vi "parse_dictionary_to_csv_string.vi"(8 "error in (no error)":errorcluster, 11 "Localization":T1) -> (0 "error out":errorcluster, 3 "CSV String":string)   [LabVIEW 2019]
uses:
  Dictionary--Cluster.ctl
  Font -- Cluster.ctl
  Phrase Dictionary Entry -- Cluster.ctl
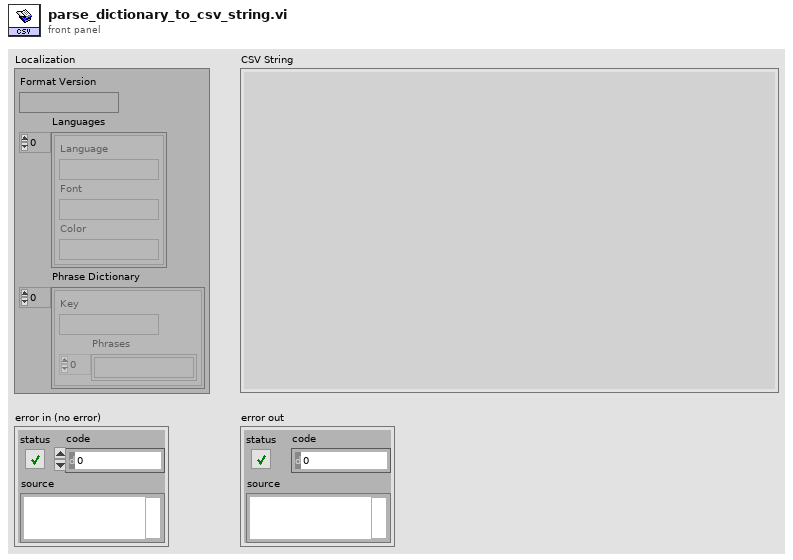
[diagram p1: front panel]
types:
  T1 = typedef "Dictionary--Cluster.ctl" = cluster{"Format Version":string, "Languages":T2[], "Phrase Dictionary":T3[]}
  T2 = typedef "Font -- Cluster.ctl" = cluster{"Language":string, "Font":string, "Color":string}
  T3 = typedef "Phrase Dictionary Entry -- Cluster.ctl" = cluster{"Key":string, "Phrases":string[]}
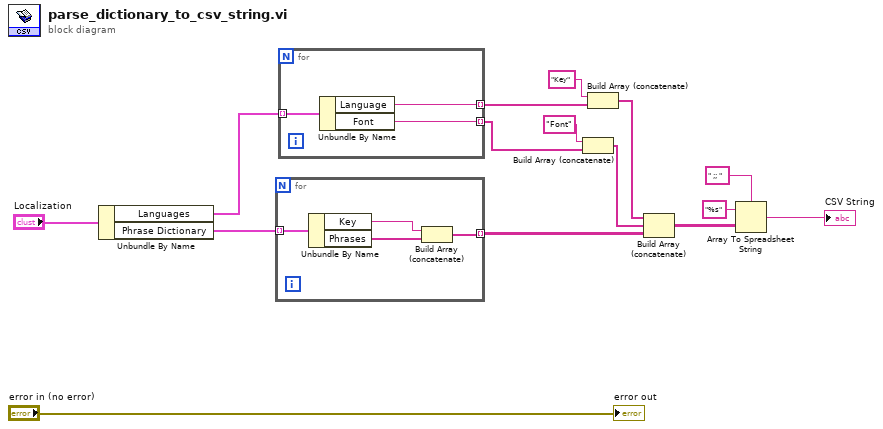
[diagram p0: block diagram]
diagram:
  n1 = Unbundle By Name("Localization") -> ("Languages"=w13:T2[], "Phrase Dictionary"=w12:T3[])
  n2 = for {
    tunnel: w12 -> [w19] mode=indexing
    tunnel: [w16] -> w11 mode=indexing
    n3 = Unbundle By Name(w19) -> ("Key"=w18:string, "Phrases"=w17:string[])
    n4 = Build Array (concatenate)(w18, w17) -> (w16:string[])
  }
  n5 = for {
    tunnel: w13 -> [w22] mode=indexing
    tunnel: [w21] -> w10 mode=indexing
    tunnel: [w20] -> w5 mode=indexing
    n6 = Unbundle By Name(w22) -> ("Language"=w21:string, "Font"=w20:string)
  }
  n7 = Build Array (concatenate)("Font", w5) -> (w6:string[])
  n8 = Build Array (concatenate)("Key", w10) -> (w9:string[])
  n9 = Build Array (concatenate)(w9, w6, w11) -> (w4:string[][])
  n10 = Array To Spreadsheet String(delimiter (Tab)=" ;; ", array=w4, 3:"%s" ("format string")) -> (spreadsheet string=→"CSV String":string)
  "error out" <- "error in (no error)"
